vi "Add Queue To Registry.vi"(0 "message queue in":T1, 5 "name":string, 11 "error in":errorcluster) -> (4 "message queue out":T1, 15 "error out":errorcluster)   [LabVIEW 2015, in "TLB` Template.lvlib" / "AMC.lvlib"]
doc: "Adds a message queue to the queue registry.\n\nThis VI returns an error if \"name\" is empty.TLB Prime - Application Template 1.3.0.24\nNorm Kirchner, NI Systems Engineering - NI\nCopyright (c) 2014, NI"
uses:
  AMC.lvlib
  Message Queue.ctl
  Message.ctl
  KeyedArray.ctl
  Queue Registry Method.ctl
  Queue Registry Properties.ctl
  Tools_KeyedArray.lvlib
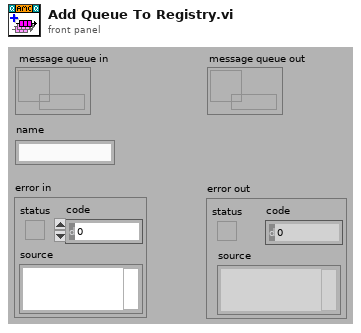
[diagram p1: front panel]
types:
  T1 = typedef "TLB` Template.lvlib/AMC.lvlib/Message Queue.ctl" = refnum<queue>
  T2 = typedef "TLB` Template.lvlib/AMC.lvlib/Queue Registry Properties.ctl" = cluster{"Name":string}
  T3 = typedef "TLB` Template.lvlib/AMC.lvlib/Queue Registry Method.ctl" = enum16{"Initialize", "Add Queue", "Set Properties", "Get Queue by Index", "Get Queue by Name", "Remove Queue", "Remove All Queues"}
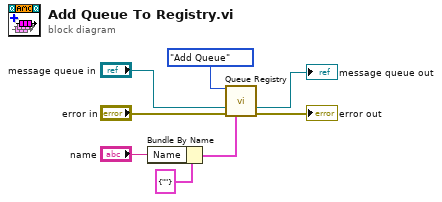
[diagram p0: block diagram]
diagram:
  n1 = Bundle By Name(cluster=T2 {"Name"=""} ("Properties In"), "Name"="name") -> (w5:T2)
  n2 = call "Queue Registry.vi"("method"=Queue_Registry_Method."Add Queue" ("Method"), "message queue in"="message queue in", "error in"="error in", "properties in"=w5) -> ("message queue out"=→"message queue out":T1, "error out"=→"error out":errorcluster)  [unwired: 6 in, 4 out]
